vi "Send general triggers setup.vi"(8 "error in (no error)":errorcluster, 11 "Refnum in":T4) -> (0 "error out":errorcluster, 3 "Refnum out":T4)   [LabVIEW 2017]
uses:
  RIG-SPECIFIC FILES/FPGA Refs/FPGA Ref.ctl
  Typedefs/Trigger 1 selector enum.ctl
  Peripherals Control/Triggers/Typedefs/General trigger settings cluster.ctl
  FPGA Typedefs/General trig pulse width.ctl
  Typedefs/HW config states enum.ctl
  <vilib>/Utility/error.llb/Error Cluster From Error Code.vi
  <vilib>/rvi/errors/niLvFpgaAdjustHostInterfaceError.vi
  <vilib>/rvi/interface/nirviReadWriteControl/nirviReadWriteControl.xnode
  NiFpgaLv.dll
  <vilib>/rvi/interface/Simulation/niFpgaSimulationCallBeginRW.vi
panel:
  out "General trigger settings":T1={"Trigger 1 function"=enum."Encoder trigger", "Triggers loop clock (MHz)"=80.0} {"Triggers loop clock (MHz)" format="%#_13g"}
  out "PXI Trig 0 (redundant)":bool
  out "General trig. pulse width":T3={"Trigger 1 function"=enum."Encoder trigger", "Pulse width (us)-Line Trig."=1, "Pulse width (us)-Frame/Cycle Trig."=1, "Pulse width (us)-Trial trig."=1000, "Pulse width (us)-Start of Exp. trig."=1000}
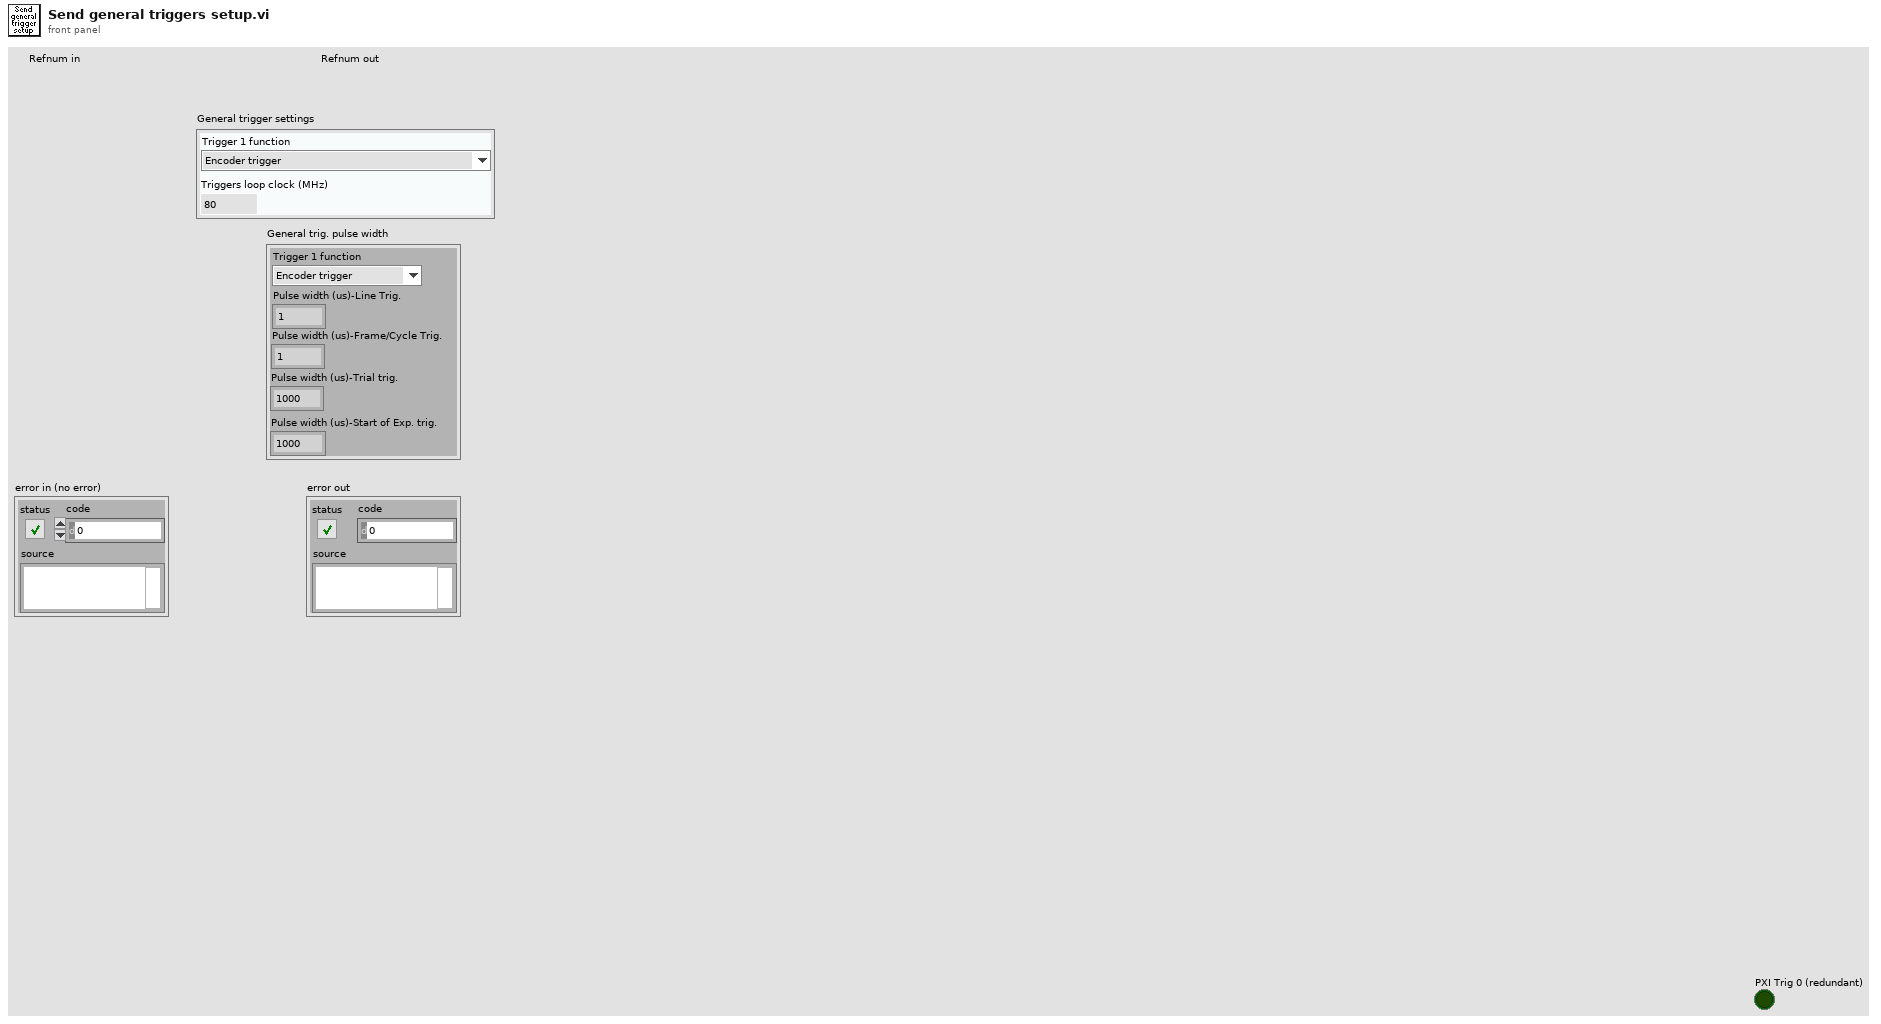
[diagram p1: front panel]
types:
  T1 = typedef "General trigger settings cluster.ctl" = cluster{"Trigger 1 function":T2, "Triggers loop clock (MHz)":dbl}
  T2 = typedef "Trigger 1 selector enum.ctl" = enum16{"Encoder trigger", "Line trigger", "Control system's ref frame acknowledgement"}
  T3 = cluster{"Trigger 1 function":T2, "Pulse width (us)-Line Trig.":u16, "Pulse width (us)-Frame/Cycle Trig.":u16, "Pulse width (us)-Trial trig.":u16, "Pulse width (us)-Start of Exp. trig.":u16}
  T4 = typedef "FPGA Ref.ctl" = refnum<k20>
  T5 = typedef "HW config states enum.ctl" = enum16{"Load from file", "Save to file", "Write all", "Read all", "Write XY stage settings", "Write DAQ FPGA settings", "Write Control FPGA settings", "Write Phys Channels", "Write System Config", "Write HW Config", "Save System Config", "Save HW Config", "Clear", "Compare from file"}
  T6 = typedef "General trig pulse width.ctl" = cluster{"Trigger 1 function":T2, "Pulse width (ticks)-Line Trig.":u32, "Pulse width (ticks)-Frame/Cycle Trig.":u32, "Pulse width (ticks)-Trial trig.":u32, "Pulse width (ticks)-Start of Exp. trig.":u32}
  T7 = typedef "Triggers output setup.ctl" = T8[]
  T8 = typedef "Trigger setup element cluster.ctl" = cluster{"Name":string, "Output?":bool, "Output terminal":tag, "PXI backplane line":tag, "Pulse width (us)":u16}
  T9 = cluster{"Enable Trigger 1":bool, "Enable Trigger 2":bool, "Enable Trigger 3":bool, "Enable Trigger 4":bool}
  T10 = cluster{"[0]":u16, "[1]":u16, "[2]":u16, "[3]":u16, "[4]":u16, "[5]":u16, "[6]":u16, "[7]":u16, "[8]":u16}
  T11 = cluster{"Trigger 1 function":T2, "[1]":u16, "[2]":u16, "[3]":u16, "[4]":u16}
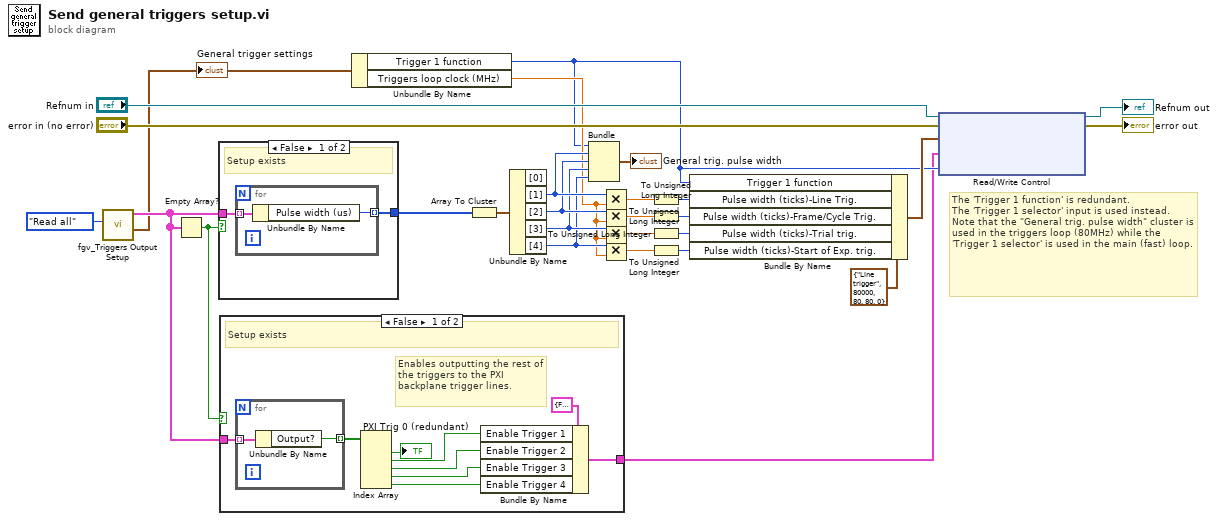
[diagram p0: block diagram]
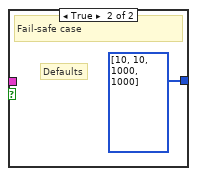
[diagram p3: hidden frame]
diagram:
  # "The 'Trigger 1 function' is redundant.\nThe 'Trigger 1 selector' input is used instead.\nNote that the \"General trig. pulse width\" cluster is used in the triggers loop (80MHz) while the  'Trigger 1 selector' is used in the main (fast) loop."
  n1 = call "fgv_Triggers Output Setup.vi"("Function"=HW_config_states_enum."Read all") -> ("General trigger settings"=w3:T1, "Triggers output setup"=w6:T7)  [unwired: 8 in, 1 out]
  "General trigger settings" <- w3
  n2 = Empty Array?(array=w6) -> (empty?=w5:bool)
  n3 = case shown="False" w5 {
    tunnel: w6 -> [w30 _]
    tunnel: [w29 u16[] [10, 10, 1000, 1000]] -> w14
    frame False {
      # "Setup exists"
      n4 = for {
        tunnel: w30 -> [w32] mode=indexing
        tunnel: [w31] -> w29 mode=indexing
        n5 = Unbundle By Name(w32) -> ("Pulse width (us)"=w31:u16)
      }
    }
    frame True {
      # "Defaults"
      # "Fail-safe case"
    }
  }
  n6 = case shown="False" w5 {
    tunnel: [w36 _] -> w1
    tunnel: w6 -> [w35 _]
    frame False {
      # "Enables outputting the rest of the triggers to the PXI backplane trigger lines."
      # "Setup exists"
      n7 = for {
        tunnel: w35 -> [w44] mode=indexing
        tunnel: [w43] -> w42 mode=indexing
        n8 = Unbundle By Name(w44) -> ("Output?"=w43:bool)
      }
      n9 = Index Array(array=w42) -> (element #1=→"PXI Trig 0 (redundant)":bool, element #2=w41:bool, element #3=w40:bool, element #4=w39:bool, element #5=w38:bool)  [unwired: 5 in]
      n10 = Bundle By Name(cluster=T9 {"Enable Trigger 1"=FALSE, "Enable Trigger 2"=FALSE, "Enable Trigger 3"=FALSE, "Enable Trigger 4"=FALSE} ("PXI Trigger Enable"), "Enable Trigger 1"=w41, "Enable Trigger 2"=w40, "Enable Trigger 3"=w39, "Enable Trigger 4"=w38) -> (w36:T9)
    }
    frame True {
      # "Fail-safe case"
    }
  }
  n11 = Unbundle By Name(w3) -> ("Trigger 1 function"=w2:T2, "Triggers loop clock (MHz)"=w4:dbl)
  n12 = Array To Cluster(array=w14) -> (cluster=w13:T10)
  n13 = Unbundle By Name(w13) -> ("[1]"=w12:u16, "[2]"=w11:u16, "[3]"=w10:u16, "[4]"=w9:u16)  [unwired: 1 out]
  n14 = Bundle("Trigger 1 function"=w2, "[1]"=w12, "[2]"=w11, "[3]"=w10, "[4]"=w9) -> (→"General trig. pulse width":T11)  [unwired: 1 in]
  n15 = Multiply(x=w12, y=w4) -> (x*y=w24:dbl)
  n16 = Multiply(x=w11, y=w4) -> (x*y=w21:dbl)
  n17 = Multiply(x=w10, y=w4) -> (x*y=w18:dbl)
  n18 = Multiply(x=w9, y=w4) -> (x*y=w17:dbl)
  n19 = To Unsigned Long Integer(number=w24) -> (unsigned 32bit integer=w22:u32)
  n20 = To Unsigned Long Integer(number=w21) -> (unsigned 32bit integer=w20:u32)
  n21 = To Unsigned Long Integer(number=w18) -> (unsigned 32bit integer=w19:u32)
  n22 = To Unsigned Long Integer(number=w17) -> (unsigned 32bit integer=w16:u32)
  n23 = Bundle By Name(cluster=T6 {"Trigger 1 function"=enum."Line trigger", "Pulse width (ticks)-Line Trig."=80000, "Pulse width (ticks)-Frame/Cycle Trig."=80, "Pulse width (ticks)-Trial trig."=80, "Pulse width (ticks)-Start of Exp. trig."=0} ("General trig. pulse width"), "Trigger 1 function"=w2, "Pulse width (ticks)-Line Trig."=w22, "Pulse width (ticks)-Frame/Cycle Trig."=w20, "Pulse width (ticks)-Trial trig."=w19, "Pulse width (ticks)-Start of Exp. trig."=w16) -> (w23:T6)
  n24 = xnode ("Read/Write Control")("FPGA VI Reference In"="Refnum in", "error in"="error in (no error)", "General trig. pulse width"=w23, "PXI Trigger Enable"=w1, "Trigger 1 selector"=w2) -> ("FPGA VI Reference Out"=→"Refnum out":T4, "error out"=→"error out":errorcluster)
